vi "dfd_Calculate Element Matrix Positions.vi"(4 "Height Gap":u32, 6 "Width Gap":u32, 9 "origin":cluster{"x":i16, "y":i16}, 11 "Object Bounds":cluster{"Width":u32, "Height":u32}[][](array[cluster])=[[{"Width"=0, "Height"=19}, {"Width"=75, "Height"=34}]]) -> (1 "Right Bracket":cluster{"x":u32, "y":u32}[](array[cluster])=[{"x"=82, "y"=20}, {"x"=85, "y"=20}, {"x"=85, "y"=54}, {"x"=82, "y"=54}], 2 "Left Bracket":cluster{"x":i16, "y":u32}[](array[cluster])=[{"x"=13, "y"=20}, {"x"=10, "y"=20}, {"x"=10, "y"=54}, {"x"=13, "y"=54}], 3 "Origins Position":cluster{"x":i16, "y":i16}[][](array[cluster])=[[{"x"=10, "y"=28}, {"x"=10, "y"=20}]], 5 "rect":T1={"left"=0, "top"=0, "right"=75, "bottom"=34})   [LabVIEW 2017, in "NI_DigFilter_Process.lvlib"]
uses:
  <vilib>/addons/Digital Filter Design/NI_DigFilter_Process.lvlib
panel:
  out "Max Column":cluster{"Width":u32, "Height":u32}[](array[cluster])=[{"Width"=0, "Height"=19}, {"Width"=75, "Height"=34}]
  out "Max Row":cluster{"Width":u32, "Height":u32}[](array[cluster])=[{"Width"=75, "Height"=34}]
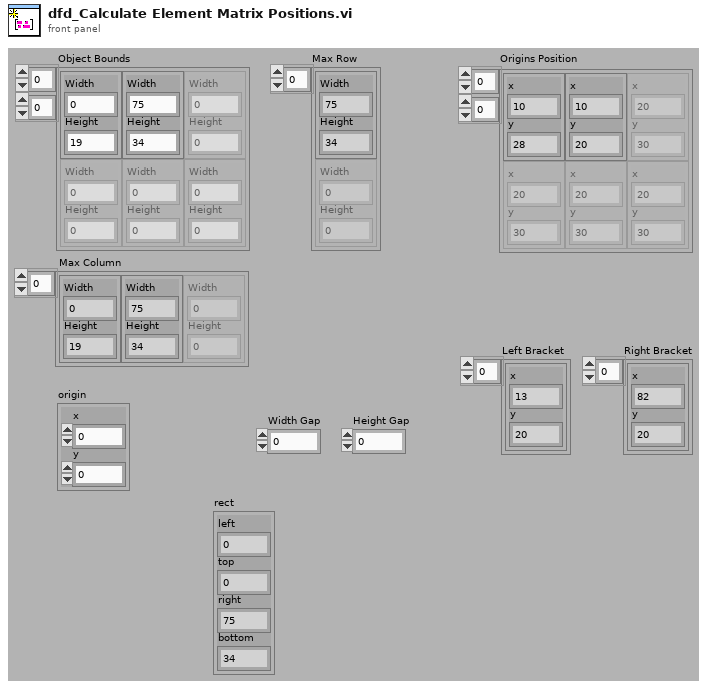
[diagram p1: front panel]
types:
  T1 = cluster{"left":i16, "top":i16, "right":i16, "bottom":i16}
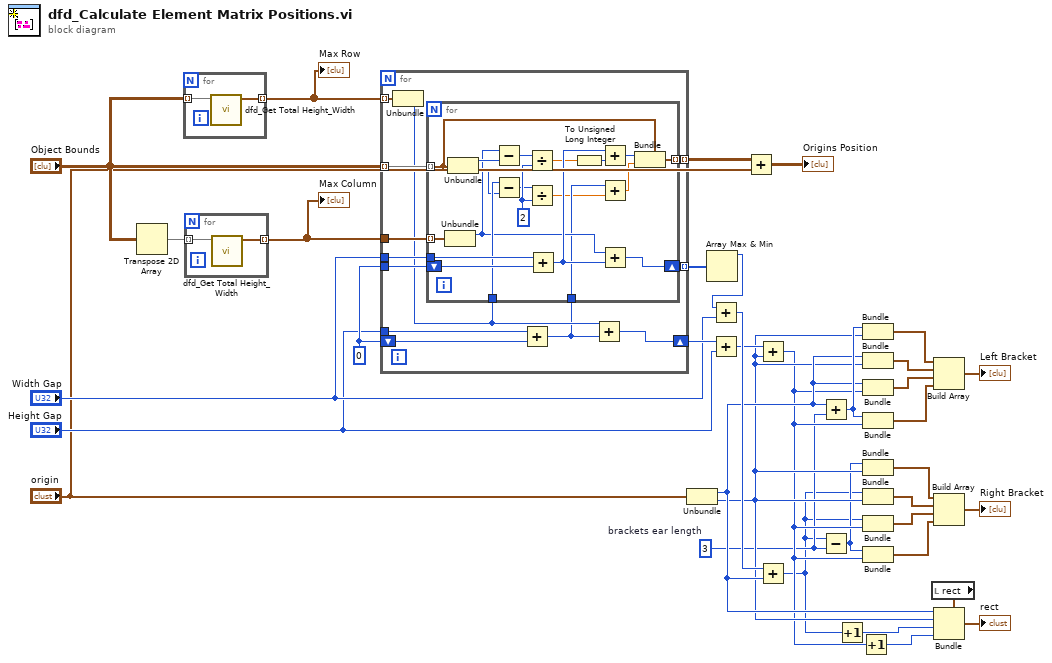
[diagram p0: block diagram]
diagram:
  w13 = u32 3  # brackets ear length
  w22 = u32 0
  n1 = Transpose 2D Array(2D array="Object Bounds") -> (transposed array=w19:cluster{"Width":u32, "Height":u32}[][])
  n2 = for {
    tunnel: "Object Bounds" -> [w38] mode=indexing
    tunnel: [w37] -> w8 mode=indexing
    n3 = call <vilib>:"dfd_Get Total Height_Width.vi"("Array"=w38) -> ("Bounds"=w37:cluster{"Width":u32, "Height":u32})  [unwired: 10 out]
  }
  "Max Row" <- w8
  n4 = for {
    tunnel: w19 -> [w40] mode=indexing
    tunnel: [w39] -> w21 mode=indexing
    n5 = call <vilib>:"dfd_Get Total Height_Width.vi"("Array"=w40) -> ("Bounds"=w39:cluster{"Width":u32, "Height":u32})  [unwired: 10 out]
  }
  "Max Column" <- w21
  n6 = for {
    tunnel: "Object Bounds" -> [w52] mode=indexing
    tunnel: w8 -> [w45] mode=indexing
    tunnel: w21 -> [w48]
    tunnel: "Width Gap" -> [w51]
    tunnel: w22 -> [w50]
    shift-right: [w47] -> w23
    shift-left: w22 -> [w49]
    tunnel: "Height Gap" -> [w43]
    tunnel: [w46] -> w10 mode=indexing
    tunnel: [w41] -> w2 mode=indexing
    n7 = Unbundle(w45) -> ("Height"=w44:u32)  [unwired: 1 out]
    n8 = Add(x=w43, y=w49) -> (x+y=w42:u32)
    n9 = for {
      tunnel: w52 -> [w64] mode=indexing
      tunnel: w48 -> [w70] mode=indexing
      tunnel: w51 -> [w72]
      shift-right: [w67] -> w41
      shift-left: w50 -> [w69]
      tunnel: w42 -> [w55]
      tunnel: w44 -> [w63]
      tunnel: [w71] -> w46 mode=indexing
      w57 = u32 2 ("y")
      n10 = Unbundle(w70) -> ("Width"=w60:u32)  [unwired: 1 out]
      n11 = Unbundle(w64) -> ("Width"=w61:u32, "Height"=w62:u32)
      n12 = Subtract(x=w60, y=w61) -> (x-y=w59:u32)
      n13 = Subtract(x=w63, y=w62) -> (x-y=w56:u32)
      n14 = Divide(x=w59, y=w57) -> (x/y=w58:dbl)
      n15 = Divide(x=w56, y=w57) -> (x/y=w53:dbl)
      n16 = Add(x=w72, y=w69) -> (x+y=w68:u32)
      n17 = To Unsigned Long Integer(number=w58) -> (unsigned 32bit integer=w54:u32)
      n18 = Add(x=w68, y=w54) -> (x+y=w65:u32)
      n19 = Add(x=w55, y=w53) -> (x+y=w66:dbl)
      n20 = Add(x=w60, y=w68) -> (x+y=w67:u32)
      n21 = Bundle(cluster=w64, "Width"=w65, "Height"=w66) -> (w71:cluster{"Width":u32, "Height":u32})
    }
    n22 = Add(x=w44, y=w42) -> (x+y=w47:u32)
  }
  n23 = Unbundle("origin") -> ("x"=w16:i16, "y"=w15:i16)
  n24 = Array Max & Min(array=w2) -> (max value=w1:u32)  [unwired: 3 out]
  n25 = Add(x=w1, y="Width Gap") -> (x+y=w36:u32)
  n26 = Add(x=w23, y="Height Gap") -> (x+y=w35:u32)
  n27 = Add(x=w10, y="origin") -> (x+y=→"Origins Position":cluster{u32, u32}[][])
  n28 = Add(x=w35, y=w15) -> (x+y=w14:u32)
  n29 = Add(x=w36, y=w16) -> (x+y=w11:u32)
  n30 = Add(x=w16, y=w13) -> (x+y=w29:u32)
  n31 = Subtract(x=w11, y=w13) -> (x-y=w12:u32)
  n32 = Increment(x=w11) -> (x+1=w4:u32)
  n33 = Increment(x=w14) -> (x+1=w3:u32)
  n34 = Bundle(w29, "y"=w15) -> (w24:cluster{u32, "y":i16})  [unwired: 1 out]
  n35 = Bundle("x"=w16, "y"=w15) -> (w25:cluster{"x":i16, "y":i16})  [unwired: 1 out]
  n36 = Bundle("x"=w16, w14) -> (w26:cluster{"x":i16, u32})  [unwired: 1 out]
  n37 = Bundle(w29, w14) -> (w27:cluster{u32, u32})  [unwired: 1 out]
  n38 = Bundle(w12, "y"=w15) -> (w33:cluster{u32, "y":i16})  [unwired: 1 out]
  n39 = Bundle(w11, "y"=w15) -> (w32:cluster{u32, "y":i16})  [unwired: 1 out]
  n40 = Bundle(w11, w14) -> (w31:cluster{u32, u32})  [unwired: 1 out]
  n41 = Bundle(w12, w14) -> (w30:cluster{u32, u32})  [unwired: 1 out]
  n42 = local read "rect"() -> (w17:T1)
  n43 = Build Array(w24, w25, w26, w27) -> (→"Left Bracket":cluster{"x":u32, "y":u32}[])
  n44 = Build Array(w33, w32, w31, w30) -> (→"Right Bracket":cluster{u32, "y":u32}[])
  n45 = Bundle(cluster=w17, "left"=w16, "top"=w15, "right"=w4, "bottom"=w3) -> (→"rect":T1)
